vi "Template Pattern - Display.vi"(8 "error in (no error)":errorcluster, 11 "PopUp in":refnum<class "Popup.lvclass">) -> (0 "error out":errorcluster, 3 "PopUp out":refnum<class "Popup.lvclass">)   [LabVIEW 2021, in "Pop-Up.lvlib" / "Popup.lvclass"]
doc: "A \"Template Pattern\" VI that will call the display child for the given pop-up type and set up/tear down the pre-empt messaging\n\n<b>Code Developed By:</b>\nDaniel Coons\nTechnology Service Corporation\n1983 S Liberty Drive\nBloomington, IN 47403\nPhone: 812 558-7100\ndaniel.coons@tsc.com\nwww.tsc.com/atcs"
uses:
  Popup.lvclass
  Popup.lvclass/Popup.ctl
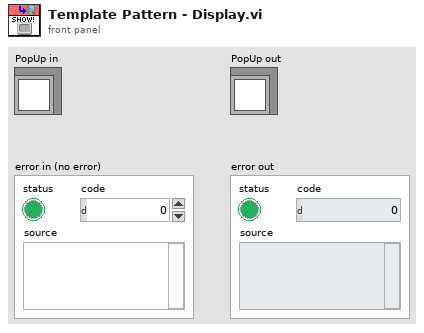
[diagram p1: front panel]
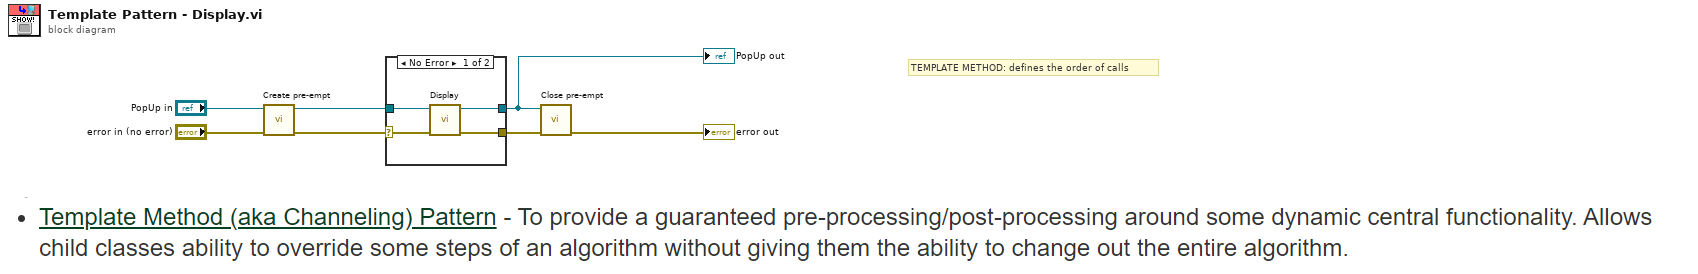
[diagram p0: block diagram]
diagram:
  # "TEMPLATE METHOD: defines the order of calls"
  n1 = call "Create pre-empt.vi"("error in (no error)"="error in (no error)", "_Popup in"="PopUp in") -> ("error out"=w3:errorcluster, "_Popup out"=w5:refnum<class "Popup.lvclass">)  [unwired: 8 in]
  n2 = case shown="No Error" w3 {
    selector: w3 -> [w8 w13]
    tunnel: w5 -> [w11 w12]
    tunnel: [w10 w12] -> w7
    tunnel: [w9 w13] -> w2
    frame No Error {
      n3 = call-dynamic "Display.vi"("error in"=w8, "Popup in"=w11) -> ("error out"=w9:errorcluster, "Popup out"=w10:refnum<class "Popup.lvclass">)  [unwired: 8 in]
    }
    frame Error {
    }
  }
  "PopUp out" <- w7
  n4 = call "Close pre-empt.vi"("error in (no error)"=w2, "_Popup in"=w7) -> ("error out"=→"error out":errorcluster)  [unwired: 9 in]
